vi "DescriptReceivedMsg SingleBoard (SubVI).vi"(8 "error constant":errorcluster, 11 "RxMessageArray":u8[](array[numeric]) format="%.0x") -> (0 "error constant":errorcluster, 3 "DataMessage Rx":T1={"Data"="", "idx"=0, "DataType"=enum."Int", "Cmd id"=200, "Get/Set"=enum."Set"})   [LabVIEW 2017]
panel:
  out "Cmd ID":u16
  out "DataReceiveFloat":sgl
  out "Float(T)Int(F)":bool
  out "DataReceiveInt":i32
  out "Index":u8
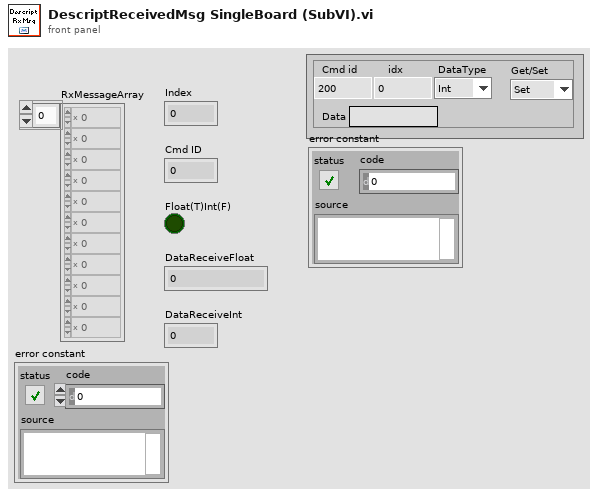
[diagram p1: front panel]
types:
  T1 = cluster{"Data":string, "idx":u16, "DataType":enum8{"Int", " float"}, "Cmd id":u16, "Get/Set":enum8{"Set", "Get"}}
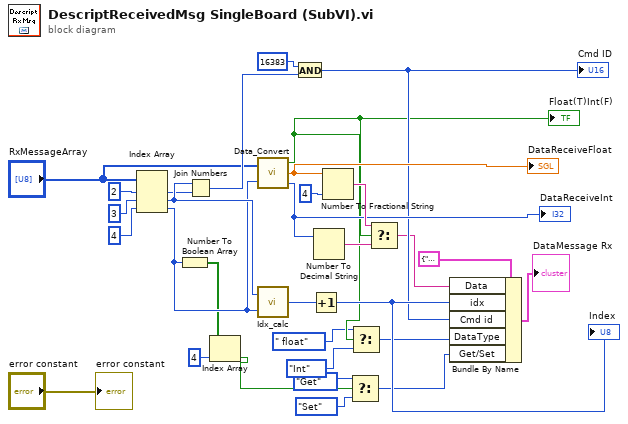
[diagram p0: block diagram]
diagram:
  n1 = Index Array(array="RxMessageArray", index #1=2 ("index"), index #2=3 ("index"), index #3=4 ("index")) -> (element #1=w27:u8, element #2=w30:u8, element #3=w7:u8)
  n2 = Number To Boolean Array(number=w7) -> (Boolean array=w6:bool[])
  n3 = Join Numbers(hi=w30, lo=w27) -> ((hi.lo)=w28:u16)
  n4 = Index Array(array=w6, index=4) -> (element=w4:bool)
  n5 = call "Data_Convert.vi"("Data Type"=w7, "Array"="RxMessageArray") -> ("D Int out"=w16:i32, "D Float out"=w21:sgl, "Int_F"=w12:bool)
  "DataReceiveInt" <- w16
  "Float(T)Int(F)" <- w12
  "DataReceiveFloat" <- w21
  n6 = call "Idx_calc.vi"("bit4"=w7, "bit3"=w30) -> ("idx"=w31:u8)
  n7 = And(x=u16 16383, y=w28) -> (x .and. y?=w15:u16)
  "Cmd ID" <- w15
  n8 = Increment(x=w31) -> (x+1=w17:u8)
  "Index" <- w17
  n9 = Number To Decimal String(number=w16) -> (decimal integer string=w18:string)  [unwired: 1 in]
  n10 = Number To Fractional String(number=w21, precision (6)=i16 4) -> (F-format string=w19:string)  [unwired: 2 in]
  n11 = Select(t=enum8{"Set", "Get"}."Get" ("Get/Set"), s=w4, f=enum8{"Set", "Get"}."Set" ("Get/Set")) -> (s? t:f=w1:enum8{"Set", "Get"})
  n12 = Select(t=enum8{"Int", " float"}." float" ("DataType"), s=w12, f=enum8{"Int", " float"}."Int" ("DataType")) -> (s? t:f=w10:enum8{"Int", " float"})
  n13 = Select(t=w19, s=w12, f=w18) -> (s? t:f=w13:string)
  n14 = Bundle By Name(cluster=T1 {"Data"="1", "idx"=0, "DataType"=enum."Int", "Cmd id"=64, "Get/Set"=enum."Set"} ("DataMessage Rx 2"), "Data"=w13, "idx"=w17, "Cmd id"=w15, "DataType"=w10, "Get/Set"=w1) -> (→"DataMessage Rx":T1)
  "error constant" <- "error constant"
